vi "XML_Write_To_File.vi"(6 "Standalone? (T)":bool=TRUE caption="独立？(T)", 8 "error in (no error)":errorcluster caption="错误输入（无错误）", 10 "XML Input":string caption="XML输入", 11 "XML File Path":path caption="XML文件路径") -> (0 "error out":errorcluster caption="错误输出", 2 "XML String":string caption="XML字符串", 3 "XML File Path(duplicate)":path caption="XML文件路径（副本）")   [LabVIEW 2018]
panel:
  out "连接的字符串":string
  in  "Prompt":string="选择XML文件路径" caption="提示"
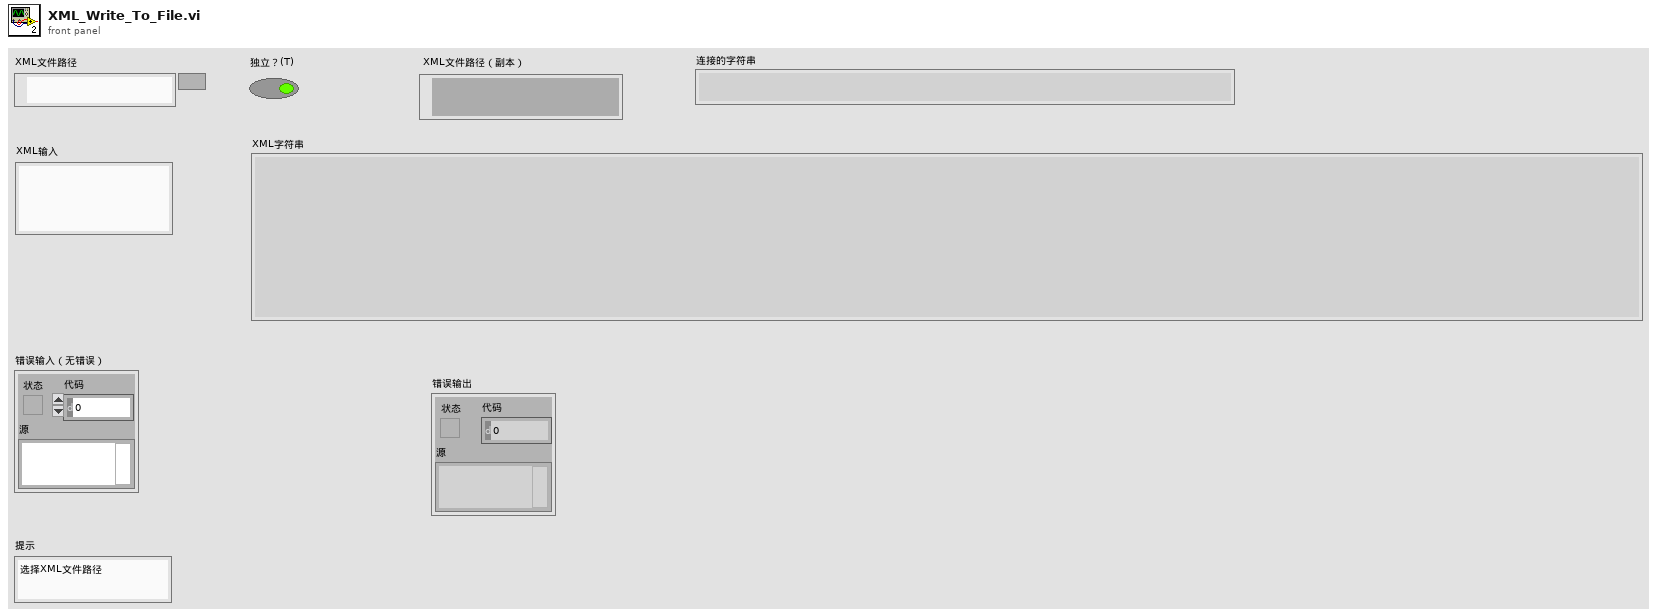
[diagram p1: front panel]
types:
  T1 = enum16{"open", "open or create", "create or replace", "create", "open (read only)"}
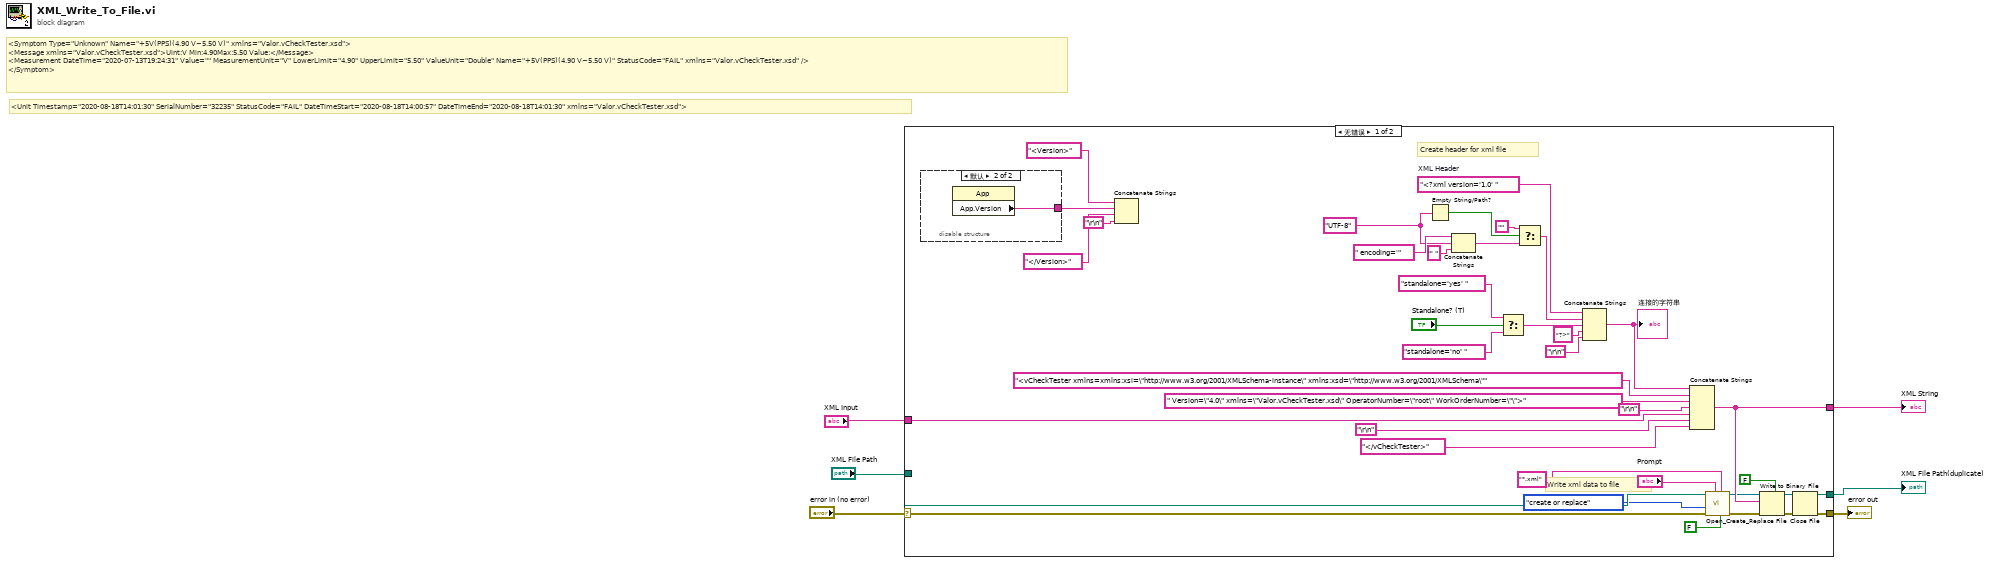
[diagram p0: block diagram]
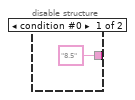
[diagram p2: hidden frame]
diagram:
  # "<Symptom Type=\"Unknown\" Name=\"+5V(PPS)(4.90 V~5.50 V)\" xmlns=\"Valor.vCheckTester.xsd\">\n<Message xmlns=\"Valor.vCheckTester.xsd\">Uint:V Min:4.90Max:5.50 Value:</Message>\n<Measurement DateTime=\"2020-07-13T19:24:31\" Value=\"\" MeasurementUnit=\"V\" LowerLimit=\"4.90\" UpperLimit=\"5.50\" ValueUnit=\"Double\" Name=\"+5V(PPS)(4.90 V~5.50 V)\" StatusCode=\"FAIL\" xmlns=\"Valor.vCheckTester.xsd\" />\n</Symptom>"
  # "<Unit Timestamp=\"2020-08-18T14:01:30\" SerialNumber=\"32235\" StatusCode=\"FAIL\" DateTimeStart=\"2020-08-18T14:00:57\" DateTimeEnd=\"2020-08-18T14:01:30\" xmlns=\"Valor.vCheckTester.xsd\">"
  n1 = case shown="无错误" "error in (no error)" {
    selector: "error in (no error)" -> [w19 w50]
    tunnel: [w20 w50] -> w3
    tunnel: "XML Input" -> [w30 w49]
    tunnel: [w18 w49] -> w4
    tunnel: [w14 w48] -> w5
    tunnel: "XML File Path" -> [w24 w48]
    frame No Error {
      w38 = "UTF-8" ("XML Encoding")
      w45 = "<?xml version='1.0' "  # XML Header
      # "Create header for xml file"
      # "Write xml data to file"
      n2 = disable-structure shown="默认" {
        disable-tunnel: ["8.5" ("App.Version") w47] -> w28
        frame condition #0 {
        }
        frame condition #1 (active) {
          n3 = property class="App"() -> ("App.Version"=w47:string)  [unwired: 2 in, 2 out]
        }
      }
      n4 = Concatenate Strings("<Version>", w28, "</Version>", "\r\n") -> ()  [unwired: 1 out]
      n5 = Empty String/Path?(string/path=w38) -> (empty?=w37:bool)
      n6 = Concatenate Strings(" encoding='", w38, "' " ("Substring")) -> (w36:string)
      n7 = Select(t="standalone='yes' " ("Substring"), s="Standalone? (T)", f="standalone='no' " ("Substring")) -> (s? t:f=w31:string)
      n8 = Select(t="", s=w37, f=w36) -> (s? t:f=w34:string)
      n9 = Concatenate Strings(w45, w34, w31, "?>" ("Substring"), "\r\n") -> (w42:string)
      "连接的字符串" <- w42
      n10 = Concatenate Strings(w42, "<vCheckTester xmlns=xmlns:xsi=\"http://www.w3.org/2001/XMLSchema-instance\" xmlns:xsd=\"http://www.w3.org/2001/XMLSchema\"" ("Substring"), " Version=\"4.0\" xmlns=\"Valor.vCheckTester.xsd\" OperatorNumber=\"root\" WorkOrderNumber=\"\">" ("字符串"), "\r\n", w30, "\r\n", "</vCheckTester>") -> (w18:string)
      n11 = call <vilib>:"Open_Create_Replace File.vi"("advisory dialog? (display:T)"=FALSE, "pattern"="*.xml", "prompt"="Prompt", "error in (no error)"=w19, "function (open:0)"=T1."create or replace", "file path"=w24) -> ("error out"=w22:errorcluster, "refnum"=w17:refnum<file>)  [unwired: 2 in, 2 out]
      n12 = Write to Binary File(file (use dialog)=w17, data=w18, error in=w22, 5:FALSE ("prepend array or string size? (T)")) -> (refnum out=w15:refnum<file>, error out=w21:errorcluster)  [unwired: 3 out]
      n13 = Close File(refnum=w15, error in=w21) -> (path=w14:path, error out=w20:errorcluster)
    }
    frame Error {
    }
  }
  "error out" <- w3
  "XML String" <- w4
  "XML File Path(duplicate)" <- w5
